vi "ORS_Alazar_acquire_multiple_frames_galvo.vi"(4 "AO.DataXferMech":i32(ring)=12590 items=["DMA"=10054, "Interrupts"=10204, "Programmed I/O"=10264, "USB Bulk"=12590], 6 "Channel":u32(ring)=1 items=["A"=1, "B"=2, "A + B"=3, "C"=4, "A + C"=5, "A + B"=6, "D"=8, "A + D"=9, "B + D"=10, "C + D"=12, "A + B + C + D"=15], 7 "Galvo":T1={"x mirror"="", "y mirror"="", "trig out"="", "x mirror task"="", "y mirror task"="", "trig out task"="", "n_axis"=0, "params"={"n_lines"=512, "n_frames"=1, "force to zero"=FALSE, "Triggers_per_sweep"=0.0, "X center"=0.0, "X span"=0.0, "Y center"=0.0, "Y span"=0.0, "flyb.lines"=0, "n_triggers"=0, "mode"=0, "offset"=5.0, "galvo phase"=0, "span factor"=1.0, "Custom trig."={"n_f to c. trig"=150, "c. trig length"=8, "c. trig interval"=1024, "n_c. trig"=1}, "f_per_pos"=1, "n_dataset"=1, "flyback fr"=1}, "acq trig out"="", "acq trig out task"="", "sample array X"=[], "sample array Y"=[], "custom trig out"="Dev1/port0/line7", "custom trig out task"="", "FDML-box"="TCPIP0::10.153.218.51::23::SOCKET", "ACQ/Galvo"=enum."ADC/FDML", "acq trig out an task"="", "acq trig out an"="", "Galvo Trig input"="", "Galvo Clk input"="", "sample array Acq trig out an"=[]} {"params"."n_dataset" min=1; "params"."X center" format="%^_3g"; "params"."X span" format="%^_3g"; "params"."Y center" format="%^_3g"; "params"."Y span" format="%^_3g"}, 8 "use_digi_trig":bool=TRUE, 9 "frame length":u32=8192, 10 "# frames":u32=10, 11 "ATSHandle":u32[](array[numeric])) -> (0 "Averaged Output":dbl[](array[numeric]), 1 "RawOutputs":i16[][](array[numeric]), 5 "Galvo out":T1={"x mirror"="", "y mirror"="", "trig out"="", "x mirror task"="", "y mirror task"="", "trig out task"="", "n_axis"=0, "params"={"n_lines"=512, "n_frames"=1, "force to zero"=FALSE, "Triggers_per_sweep"=0.0, "X center"=0.0, "X span"=0.0, "Y center"=0.0, "Y span"=0.0, "flyb.lines"=0, "n_triggers"=0, "mode"=0, "offset"=5.0, "galvo phase"=0, "span factor"=1.0, "Custom trig."={"n_f to c. trig"=150, "c. trig length"=8, "c. trig interval"=1024, "n_c. trig"=1}, "f_per_pos"=1, "n_dataset"=1, "flyback fr"=1}, "acq trig out"="", "acq trig out task"="", "sample array X"=[], "sample array Y"=[], "custom trig out"="Dev1/port0/line7", "custom trig out task"="", "FDML-box"="TCPIP0::10.153.218.51::23::SOCKET", "ACQ/Galvo"=enum."ADC/FDML", "acq trig out an task"="", "acq trig out an"="", "Galvo Trig input"="", "Galvo Clk input"="", "sample array Acq trig out an"=[]} {"params"."n_dataset" min=1; "params"."X center" format="%^_3g"; "params"."X span" format="%^_3g"; "params"."Y center" format="%^_3g"; "params"."Y span" format="%^_3g"})   [LabVIEW 2021]
uses:
  Typedefs/ORS_Galvo.ctl
  Typedefs/ORS_Galvo_params.ctl
  <vilib>/Analysis/baseanly.llb/Mean (DBL).vi
  <vilib>/Analysis/NI_AALBase.lvlib
panel:
  out "Return Code":u32=589
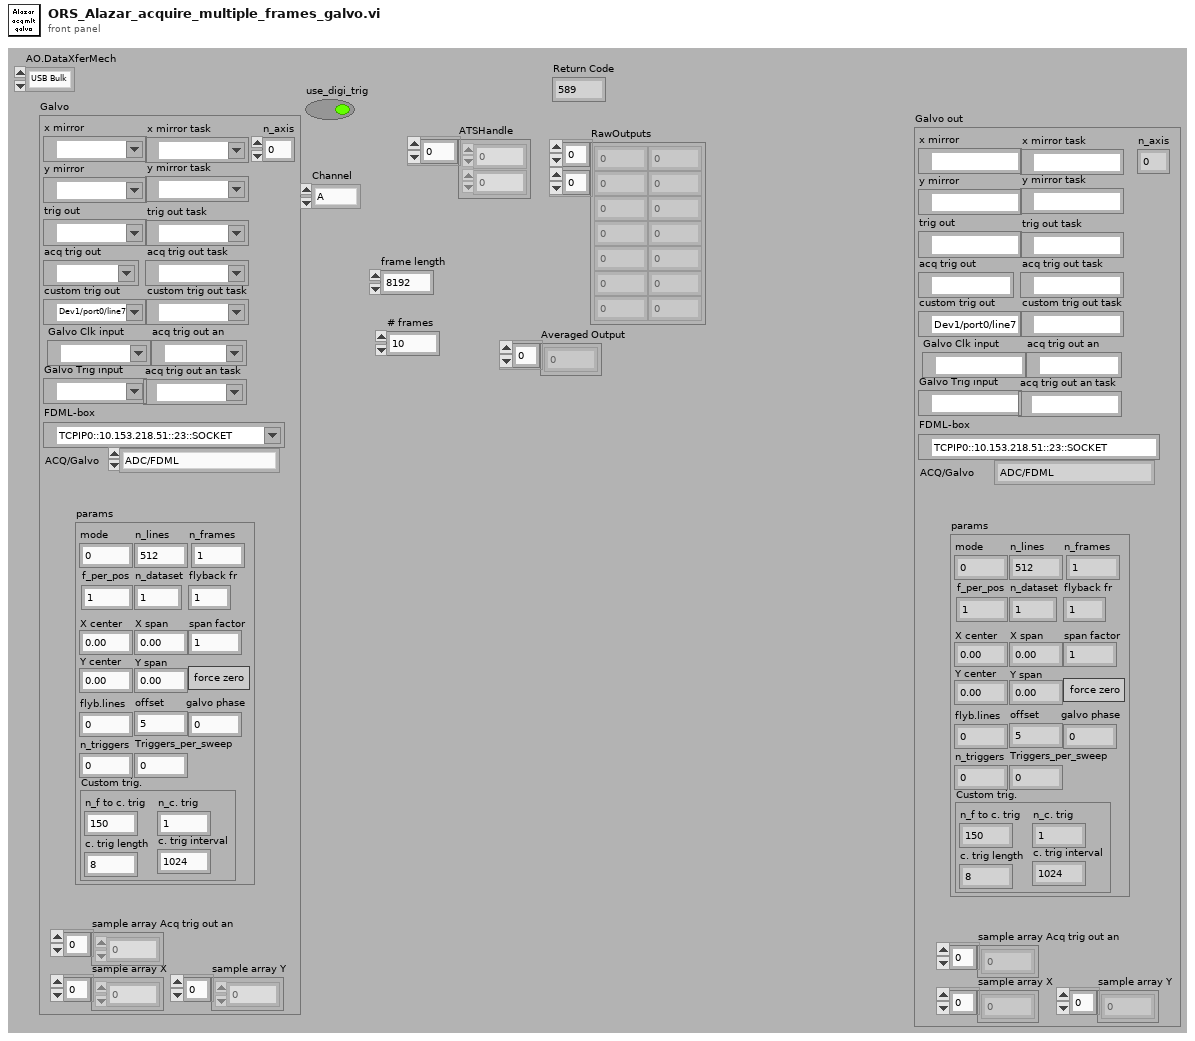
[diagram p1: front panel]
types:
  T1 = typedef "ORS_Galvo.ctl" = cluster{"x mirror":tag, "y mirror":tag, "trig out":tag, "x mirror task":refnum<k21>, "y mirror task":refnum<k21>, "trig out task":refnum<k21>, "n_axis":i32, "params":T2, "acq trig out":tag, "acq trig out task":refnum<k21>, "sample array X":dbl[], "sample array Y":dbl[], "custom trig out":tag, "custom trig out task":refnum<k21>, "FDML-box":refnum<visa-resource-name>, "ACQ/Galvo":enum16{"ADC/FDML", "NI_DAQ", "ADC"}, "acq trig out an task":refnum<k21>, "acq trig out an":tag, "Galvo Trig input":tag, "Galvo Clk input":tag, "sample array Acq trig out an":dbl[]}
  T2 = typedef "ORS_Galvo_params.ctl" = cluster{"n_lines":i32, "n_frames":i32, "force to zero":bool, "Triggers_per_sweep":dbl, "X center":dbl, "X span":dbl, "Y center":dbl, "Y span":dbl, "flyb.lines":i32, "n_triggers":i32, "mode":i32, "offset":dbl, "galvo phase":i32, "span factor":dbl, "Custom trig.":cluster{"n_f to c. trig":i32, "c. trig length":i32, "c. trig interval":i32, "n_c. trig":i32}, "f_per_pos":i32, "n_dataset":u32, "flyback fr":u16}
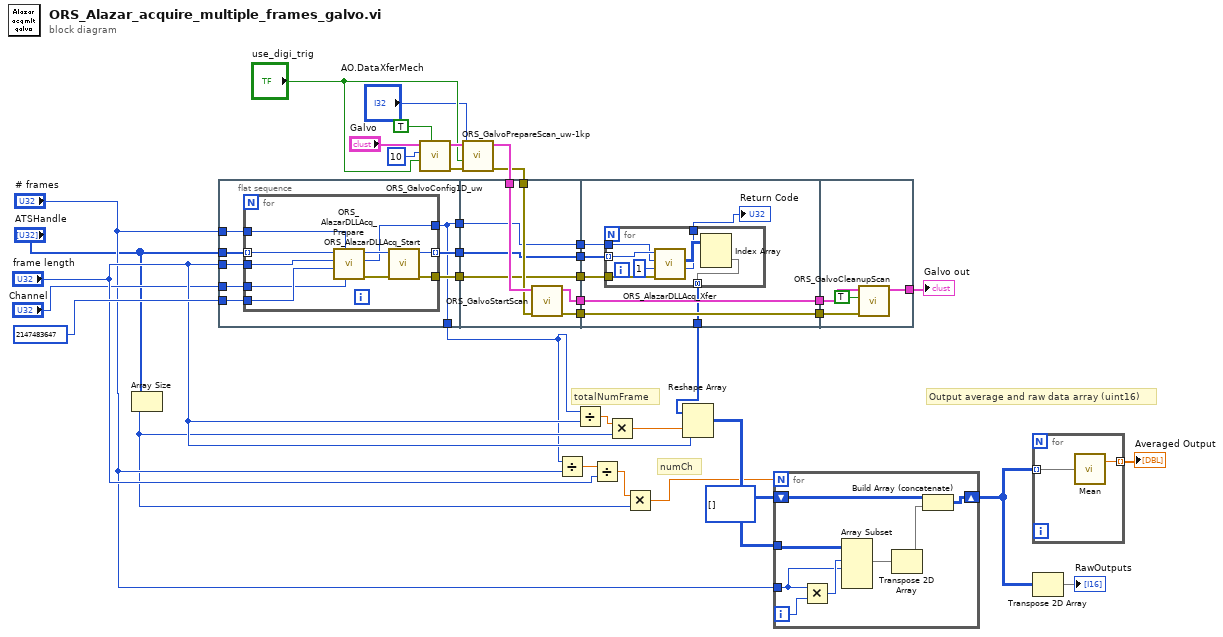
[diagram p0: block diagram]
diagram:
  # "totalNumFrame"
  # "numCh"
  # "Output average and raw data array (uint16)"
  n1 = Array Size(array="ATSHandle") -> (size(s)=w4:i32)
  n2 = flat-sequence {
    tunnel: "frame length" -> [w43]
    tunnel: "ATSHandle" -> [w46]
    tunnel: [w39] -> w35
    tunnel: [w45] -> w34
    tunnel: [w44] -> w33
    tunnel: 2147483647 ("n_triggers") -> [w42]
    tunnel: "# frames" -> [w41]
    tunnel: "Channel" -> [w40]
    tunnel: [w39] -> w3
    tunnel: w23 -> [w63]
    tunnel: w22 -> [w62]
    tunnel: [w61] -> w32
    tunnel: [w60] -> w31
    tunnel: w35 -> [w59]
    tunnel: [w59] -> w30
    tunnel: w34 -> [w58]
    tunnel: [w58] -> w29
    tunnel: [w57] -> w28
    tunnel: w33 -> [w57]
    tunnel: w32 -> [w70]
    tunnel: [w70] -> w27
    tunnel: w31 -> [w69]
    tunnel: [w69] -> w26
    tunnel: w30 -> [w65]
    tunnel: w29 -> [w68]
    tunnel: w28 -> [w67]
    tunnel: [w66] -> w2
    tunnel: w27 -> [w81]
    tunnel: w26 -> [w80]
    tunnel: [w79] -> w37
    frame #0 {
      n3 = for {
        tunnel: w46 -> [w56] mode=indexing
        tunnel: [w54] -> w39
        tunnel: [w52] -> w45 mode=indexing
        tunnel: [w51] -> w44
        tunnel: w43 -> [w50]
        tunnel: w42 -> [w49]
        tunnel: w41 -> [w48]
        tunnel: w40 -> [w47]
        n4 = call "ORS_AlazarDLLAcq_Prepare.vi"("Channel"=w47, "Records Per Buffer"=w48, "Records Count"=w49, "Record length"=w50, "ATSHandle"=w56) -> ("error out"=w53:errorcluster, "Samps Per Buffer"=w54:u32, "ATSHandle_out"=w55:u32)  [unwired: 4 in]
        n5 = call "ORS_AlazarDLLAcq_Start.vi"("error in (no error)"=w53, "ATSHandle"=w55) -> ("error out"=w51:errorcluster, "ATSHandle_out"=w52:u32)  [unwired: 8 in]
      }
    }
    frame #1 {
      n6 = call "ORS_GalvoStartScan.vi"("error in"=w62, "Galvo"=w63) -> ("error out"=w61:errorcluster, "Galvo out"=w60:T1)  [unwired: 8 in]
    }
    frame #2 {
      n7 = for {
        tunnel: w68 -> [w77] mode=indexing
        tunnel: w67 -> [w76]
        tunnel: [w72] -> w66 mode=concatenating
        tunnel: w65 -> [w74]
        tunnel: [w71] -> w64
        n8 = call "ORS_AlazarDLLAcq_Xfer.vi"("error in (no error)"=w76, "#buffers"=u32 1, "SamplesPerBuffer"=w74, "ATSHandle"=w77) -> ("Return Code"=w71:u32, "BufferArrayOut"=w73:i16[][])  [unwired: 4 in, 2 out]
        n9 = Index Array(array=w73) -> (element=w72:i16[])  [unwired: 2 in]
      }
      "Return Code" <- w64
    }
    frame #3 {
      n10 = call "ORS_GalvoCleanupScan.vi"("error in"=w81, "cleanupgalvo"=TRUE, "Galvo"=w80) -> ("Galvo out"=w79:T1)  [unwired: 7 in, 1 out]
    }
  }
  n11 = call "ORS_GalvoConfig1D_uw.vi"("Force to zero"=TRUE, "use_digi_trig"="use_digi_trig", "n_triggers"=10, "Galvo"="Galvo") -> ("error out"=w24:errorcluster, "Galvo out"=w25:T1)  [unwired: 6 in]
  n12 = call "ORS_GalvoPrepareScan_uw-1kp.vi"("error in"=w24, "use_digi_trig"="use_digi_trig", "AO.DataXferMech"="AO.DataXferMech", "Galvo"=w25) -> ("error out"=w22:errorcluster, "Galvo out"=w23:T1)  [unwired: 4 in, 2 out]
  n13 = Divide(x=w3, y="# frames") -> (x/y=w18:dbl)
  n14 = Divide(x=w3, y="frame length") -> (x/y=w8:dbl)
  n15 = Divide(x=w18, y="frame length") -> (x/y=w6:dbl)
  n16 = Multiply(x=w8, y=w4) -> (x*y=w7:dbl)
  n17 = Multiply(x=w6, y=w4) -> (x*y=w5:dbl)
  n18 = Reshape Array(w2, w7, "frame length") -> (w16:i16[][])
  n19 = for {
    N: w5 -> [_]
    tunnel: w16 -> [w89]
    shift-right: [w88] -> w13
    shift-left: i16[][] [] -> [w87]
    tunnel: "# frames" -> [w84]
    i -> [w85]
    n20 = Multiply(x=w84, y=w85) -> (x*y=w86:u32)
    n21 = Array Subset(array=w89, index (row)=w86, length (row)=w84) -> (w82:i16[][])  [unwired: 2 in]
    n22 = Transpose 2D Array(2D array=w82) -> (transposed array=w83:i16[][])
    n23 = Build Array (concatenate)(w87, w83) -> (w88:i16[][])
  }
  n24 = for {
    tunnel: w13 -> [w91] mode=indexing
    tunnel: [w90] -> w38 mode=indexing
    n25 = call-poly <vilib>:"Mean.vi"("X"=w91) -> ("mean"=w90:dbl)  [unwired: 1 out]
  }
  "Averaged Output" <- w38
  n26 = Transpose 2D Array(2D array=w13) -> (transposed array=→"RawOutputs":i16[][])
  "Galvo out" <- w37
